vi "Save UserPrefs.vi"(8 "error in (no error)":errorcluster, 11 "BluelinesRedlines in":refnum<class "BluelinesRedlines.lvclass">) -> (0 "error out":errorcluster, 3 "BluelinesRedlines out":refnum<class "BluelinesRedlines.lvclass">)   [LabVIEW 2020, in "VolatusGUIElements.lvlib" / "BluelinesRedlines.lvclass"]
uses:
  BluelinesRedlines.lvclass
  BluelinesRedlines.lvclass/BluelinesRedlines.ctl
  User BluelinesRedlines/User BluelinesRedlines.lvclass
  lv-userprefs/User Prefs/Pref Group/Pref Group.lvclass
  lv-userprefs/User Prefs/PrefsDB/PrefsDB.lvclass
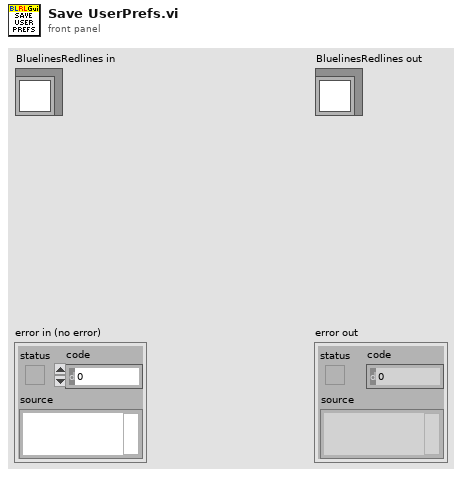
[diagram p1: front panel]
types:
  T1 = map{string, refnum<class "BluelinesRedlines Source.lvclass">}
  T2 = typedef "VolatusGUI.lvlib/BluelinesRedlines Source.lvclass/BLRL Config.ctl" = cluster{"Bluelines":T3[], "Redlines":T3[]}
  T3 = typedef "VolatusGUI.lvlib/BluelinesRedlines Source.lvclass/Range Limit Config.ctl" = cluster{"Channel":string, "Low Limit":dbl, "High Limit":dbl}
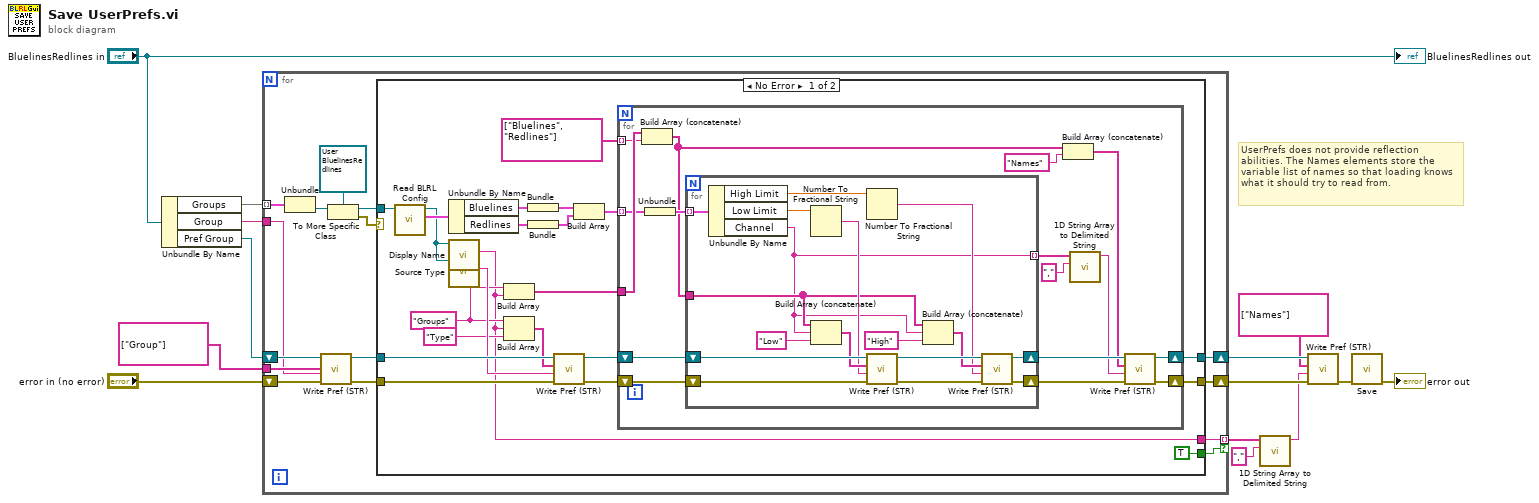
[diagram p0: block diagram]
diagram:
  # "UserPrefs does not provide reflection abilities. The Names elements store the variable list of names so that loading knows what it should try to read from."
  n1 = Unbundle By Name("BluelinesRedlines in") -> ("Groups"=w13:T1, "Group"=w11:string, "Pref Group"=w4:refnum<class "Pref Group.lvclass">)
  n2 = for {
    tunnel: w13 -> [w29] mode=indexing
    tunnel: string[] ["Group"] ("Pref Hierarchy") -> [w23]
    tunnel: w11 -> [w22]
    shift-right: [w18] -> w6
    shift-left: "error in (no error)" -> [w19]
    tunnel: [w17] -> w8 mode=indexing if=w16
    shift-right: [w15] -> w3
    shift-left: w4 -> [w24]
    n3 = Unbundle(w29) -> ("VolatusGUI:BluelinesRedlines Source.lvclass"=w28:refnum<class "BluelinesRedlines Source.lvclass">)  [unwired: 1 out]
    n4 = call "Write Pref (STR).vi"("error in (no error)"=w19, "Value"=w22, "Pref Hierarchy"=w23, "Pref Group in"=w24) -> ("error out"=w20:errorcluster, "Pref Group out"=w21:refnum<class "Pref Group.lvclass">)  [unwired: 6 in]
    n5 = To More Specific Class(target class=refnum<class "User BluelinesRedlines.lvclass"> refnum ("VolatusGUIElements.lvlib:User BluelinesRedlines.lvclass"), reference=w28) -> (specific class reference=w25:refnum<class "User BluelinesRedlines.lvclass">, error out=w26:errorcluster)  [unwired: 1 in]
    n6 = case shown="No Error" w26 {
      tunnel: w25 -> [w51 _]
      tunnel: w21 -> [w47 w85]
      tunnel: w20 -> [w46 w86]
      tunnel: [w33 w86] -> w18
      tunnel: [w32 _] -> w17
      tunnel: [TRUE _] -> w16
      tunnel: [w30 w85] -> w15
      frame No Error {
        w36 = "Groups" ("String")
        n7 = call-dynamic "Read BLRL Config.vi"("User BluelinesRedlines in"=w51) -> ("BLRL Config"=w50:T2, "User BluelinesRedlines out"=w48:refnum<class "User BluelinesRedlines.lvclass">)  [unwired: 8 in, 1 out]
        n8 = Unbundle By Name(w50) -> ("Bluelines"=w49:T3[], "Redlines"=w43:T3[])
        n9 = call-dynamic "Display Name.vi"("User BluelinesRedlines in"=w48) -> ("Display Name"=w32:string)  [unwired: 10 in]
        n10 = call-dynamic "Source Type.vi"("User BluelinesRedlines in"=w48) -> ("Source Type"=w45:string)  [unwired: 10 in]
        n11 = Build Array(w36, w32) -> (w35:string[])
        n12 = Build Array(w36, w32, "Type" ("String")) -> (w44:string[])
        n13 = Bundle("Bluelines"=w49) -> (w42:cluster{"Bluelines":T3[]})  [unwired: 1 in]
        n14 = Bundle("Redlines"=w43) -> (w41:cluster{"Redlines":T3[]})  [unwired: 1 in]
        n15 = call "Write Pref (STR).vi"("error in (no error)"=w46, "Value"=w45, "Pref Hierarchy"=w44, "Pref Group in"=w47) -> ("error out"=w34:errorcluster, "Pref Group out"=w40:refnum<class "Pref Group.lvclass">)  [unwired: 6 in]
        n16 = Build Array(w42, w41) -> (w39:cluster{"Redlines":T3[]}[])
        n17 = for {
          tunnel: w39 -> [w63] mode=indexing
          tunnel: string[] ["Bluelines", "Redlines"] ("Pref Hierarchy") -> [w66] mode=indexing
          tunnel: w35 -> [w67]
          shift-right: [w52] -> w33
          shift-left: w34 -> [w64]
          shift-right: [w53] -> w30
          shift-left: w40 -> [w65]
          n18 = Build Array (concatenate)(w67, w66) -> (w57:string[])
          n19 = Unbundle(w63) -> ("Redlines"=w62:T3[])
          n20 = for {
            tunnel: w62 -> [w82] mode=indexing
            tunnel: w57 -> [w73]
            shift-right: [w70] -> w58
            shift-left: w64 -> [w83]
            shift-right: [w69] -> w59
            shift-left: w65 -> [w84]
            tunnel: [w68] -> w60 mode=indexing
            n21 = Unbundle By Name(w82) -> ("High Limit"=w77:dbl, "Low Limit"=w79:dbl, "Channel"=w68:string)
            n22 = Number To Fractional String(number=w79) -> (F-format string=w78:string)  [unwired: 3 in]
            n23 = Build Array (concatenate)(w73, w68, "Low" ("element")) -> (w80:string[])
            n24 = Number To Fractional String(number=w77) -> (F-format string=w71:string)  [unwired: 3 in]
            n25 = call "Write Pref (STR).vi"("error in (no error)"=w83, "Value"=w78, "Pref Hierarchy"=w80, "Pref Group in"=w84) -> ("error out"=w76:errorcluster, "Pref Group out"=w75:refnum<class "Pref Group.lvclass">)  [unwired: 6 in]
            n26 = Build Array (concatenate)(w73, w68, "High" ("element")) -> (w72:string[])
            n27 = call "Write Pref (STR).vi"("error in (no error)"=w76, "Value"=w71, "Pref Hierarchy"=w72, "Pref Group in"=w75) -> ("error out"=w70:errorcluster, "Pref Group out"=w69:refnum<class "Pref Group.lvclass">)  [unwired: 6 in]
          }
          n28 = Build Array (concatenate)(w57, "Names") -> (w55:string[])
          n29 = call <vilib>:"1D String Array to Delimited String.vi"("delimiter"=",", "string array"=w60) -> ("delimited string"=w54:string)  [unwired: 9 in]
          n30 = call "Write Pref (STR).vi"("error in (no error)"=w58, "Value"=w54, "Pref Hierarchy"=w55, "Pref Group in"=w59) -> ("error out"=w52:errorcluster, "Pref Group out"=w53:refnum<class "Pref Group.lvclass">)  [unwired: 6 in]
        }
      }
      frame Error {
        # "Do not care about non-user defined groups, at least yet. If we do, would probably want to change the \"Is External.vi\" to a more general \"Source Config.vi\" or similar to specify multiple values such as wanted to be persisted."
      }
    }
  }
  n31 = call <vilib>:"1D String Array to Delimited String.vi"("delimiter"=",", "string array"=w8) -> ("delimited string"=w1:string)  [unwired: 9 in]
  n32 = call "Write Pref (STR).vi"("error in (no error)"=w6, "Value"=w1, "Pref Hierarchy"=string[] ["Names"], "Pref Group in"=w3) -> ("error out"=w5:errorcluster)  [unwired: 6 in, 1 out]
  n33 = call "Save.vi"("error in (no error)"=w5) -> ("error out"=→"error out":errorcluster)  [unwired: 9 in, 1 out]
  "BluelinesRedlines out" <- "BluelinesRedlines in"
